vi "Flush Data to Log File.vi"(8 "error in (no error)":errorcluster, 10 "Data Queue":refnum<queue>, 11 "Logging Configuration":T1) -> (0 "error out":errorcluster)   [LabVIEW 2016, in "Logging.lvlib"]
doc: "Flush the data queue of any pending data and write it to the log file. Close the TDMS file reference."
uses:
  Logging.lvlib
  Logging Configuration.ctl
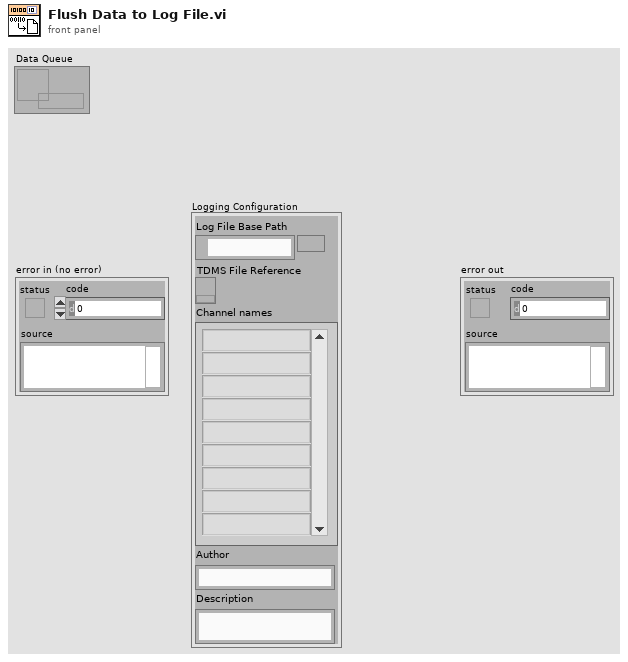
[diagram p1: front panel]
types:
  T1 = typedef "Logging.lvlib/Logging Configuration.ctl" = cluster{"Log File Base Path":path, "TDMS File Reference":refnum<k34>, "Channel names":string[], "Author":string, "Description":string}
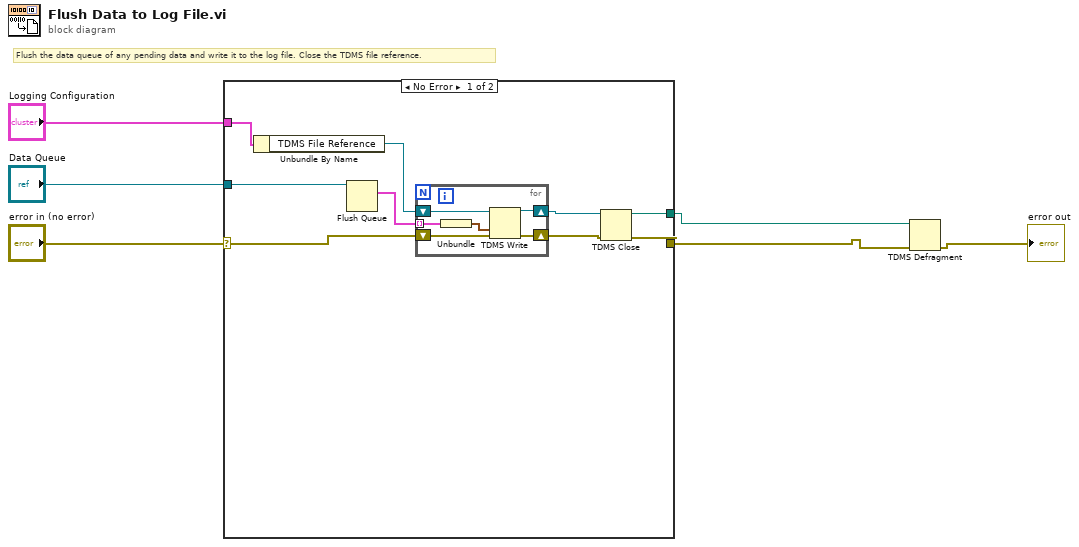
[diagram p0: block diagram]
diagram:
  # "Flush the data queue of any pending data and write it to the log file. Close the TDMS file reference."
  n1 = case shown="No Error" "error in (no error)" {
    selector: "error in (no error)" -> [w9 w22]
    tunnel: "Data Queue" -> [w12 _]
    tunnel: "Logging Configuration" -> [w11 _]
    tunnel: [w10 w22] -> w3
    tunnel: [w7 _] -> w1
    frame No Error {
      n2 = Unbundle By Name(w11) -> ("TDMS File Reference"=w13:refnum<k34>)
      n3 = Flush Queue(queue=w12) -> (remaining elements=w15:cluster{"Array":waveform(dbl)[]}[])  [unwired: 1 in, 2 out]
      n4 = for {
        shift-right: [w18] -> w8
        shift-left: w13 -> [w19]
        shift-right: [w20] -> w14
        shift-left: w9 -> [w21]
        tunnel: w15 -> [w17] mode=indexing
        n5 = Unbundle(w17) -> ("Array"=w16:waveform(dbl)[])
        n6 = TDMS Write(0:w19, 9:w16, 11:w21) -> (4:w18:refnum<k34>, 15:w20:errorcluster)  [unwired: 3 in, 2 out]
      }
      n7 = TDMS Close(8:w14, 11:w8) -> (0:w10:errorcluster, 3:w7:path)
    }
    frame Error {
    }
  }
  n8 = TDMS Defragment(4:w3, 7:w1) -> (0:→"error out":errorcluster)
